vi "G#Object_GetClassPath.vi"(0 "reference in":refnum<class "G#Interface.lvclass">, 5 "error in (no error)":errorcluster) -> (14 "reference out":refnum<class "G#Interface.lvclass">, 15 "class path":path, 19 "error out":errorcluster)   [LabVIEW 2017, in "G#Interface.lvclass"]
doc: "Returns the path to the lvclass file."
uses:
  <vilib>/addons/_AddQ/G#Interface/G#Interface.lvclass
  <vilib>/addons/_AddQ/G#Interface/G#Interface.lvclass/G#Interface.ctl
  <vilib>/addons/_AddQ/G#Object/G#Object.lvclass
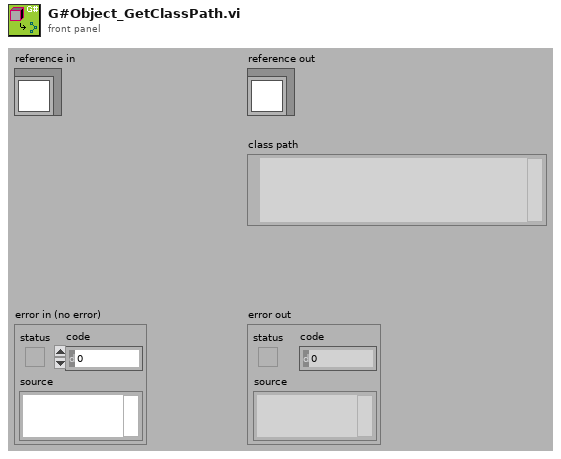
[diagram p1: front panel]
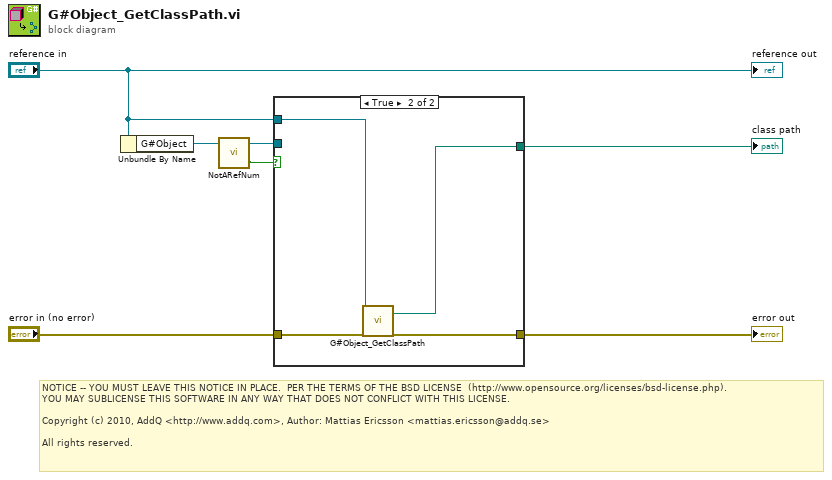
[diagram p0: block diagram]
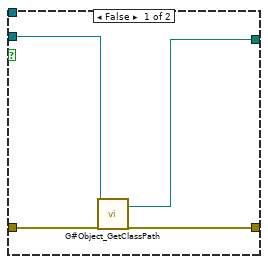
[diagram p2: hidden frame]
diagram:
  # "NOTICE -- YOU MUST LEAVE THIS NOTICE IN PLACE.  PER THE TERMS OF THE BSD LICENSE  (http://www.opensource.org/licenses/bsd-license.php).\nYOU MAY SUBLICENSE THIS SOFTWARE IN ANY WAY THAT DOES NOT CONFLICT WITH THIS LICENSE.\n\nCopyright (c) 2010, AddQ <http://www.addq.com>, Author: Mattias Ericsson <mattias.ericsson@addq.se>\n\nAll rights reserved."
  n1 = Unbundle By Name("reference in") -> ("G#Object"=w4:refnum<class "G#Object.lvclass">)
  n2 = call-dynamic "NotARefNum.vi"("reference in"=w4) -> ("not a refnum?"=w2:bool, "reference out"=w3:refnum<class "G#Object.lvclass">)  [unwired: 1 in]
  n3 = case shown="True" w2 {
    tunnel: "error in (no error)" -> [w11 w15]
    tunnel: [w10 w14] -> w6
    tunnel: [w9 w13] -> w5
    tunnel: w3 -> [w8 _]
    tunnel: "reference in" -> [_ w12]
    frame False {
      n4 = call-dynamic "G#Object_GetClassPath.vi"("reference in"=w8, "error in (no error)"=w11) -> ("class path"=w9:path, "error out"=w10:errorcluster)  [unwired: 15 in, 1 out]
    }
    frame True {
      n5 = call-parent "G#Object_GetClassPath.vi"("reference in"=w12, "error in (no error)"=w15) -> ("class path"=w13:path, "error out"=w14:errorcluster)  [unwired: 15 in, 1 out]
    }
  }
  "error out" <- w6
  "class path" <- w5
  "reference out" <- "reference in"
